vi "Read Script.vi"(2 "commands":string, 3 "script name":string) -> (0 "text from file":string, 1 "output array":dbl[][](array[numeric]))   [LabVIEW 2014]
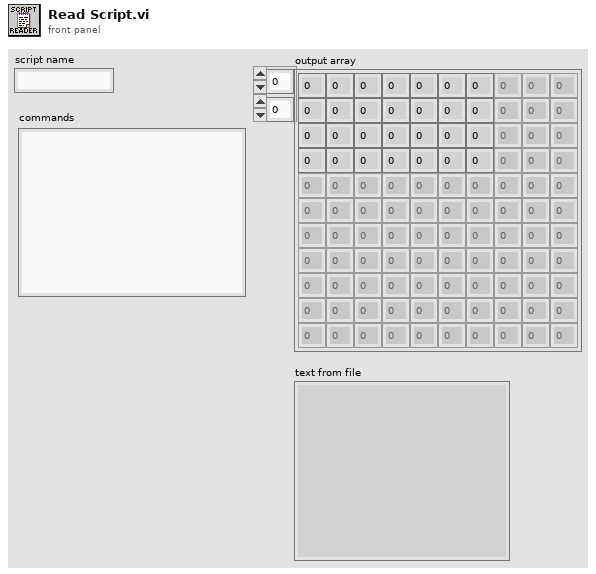
[diagram p1: front panel]
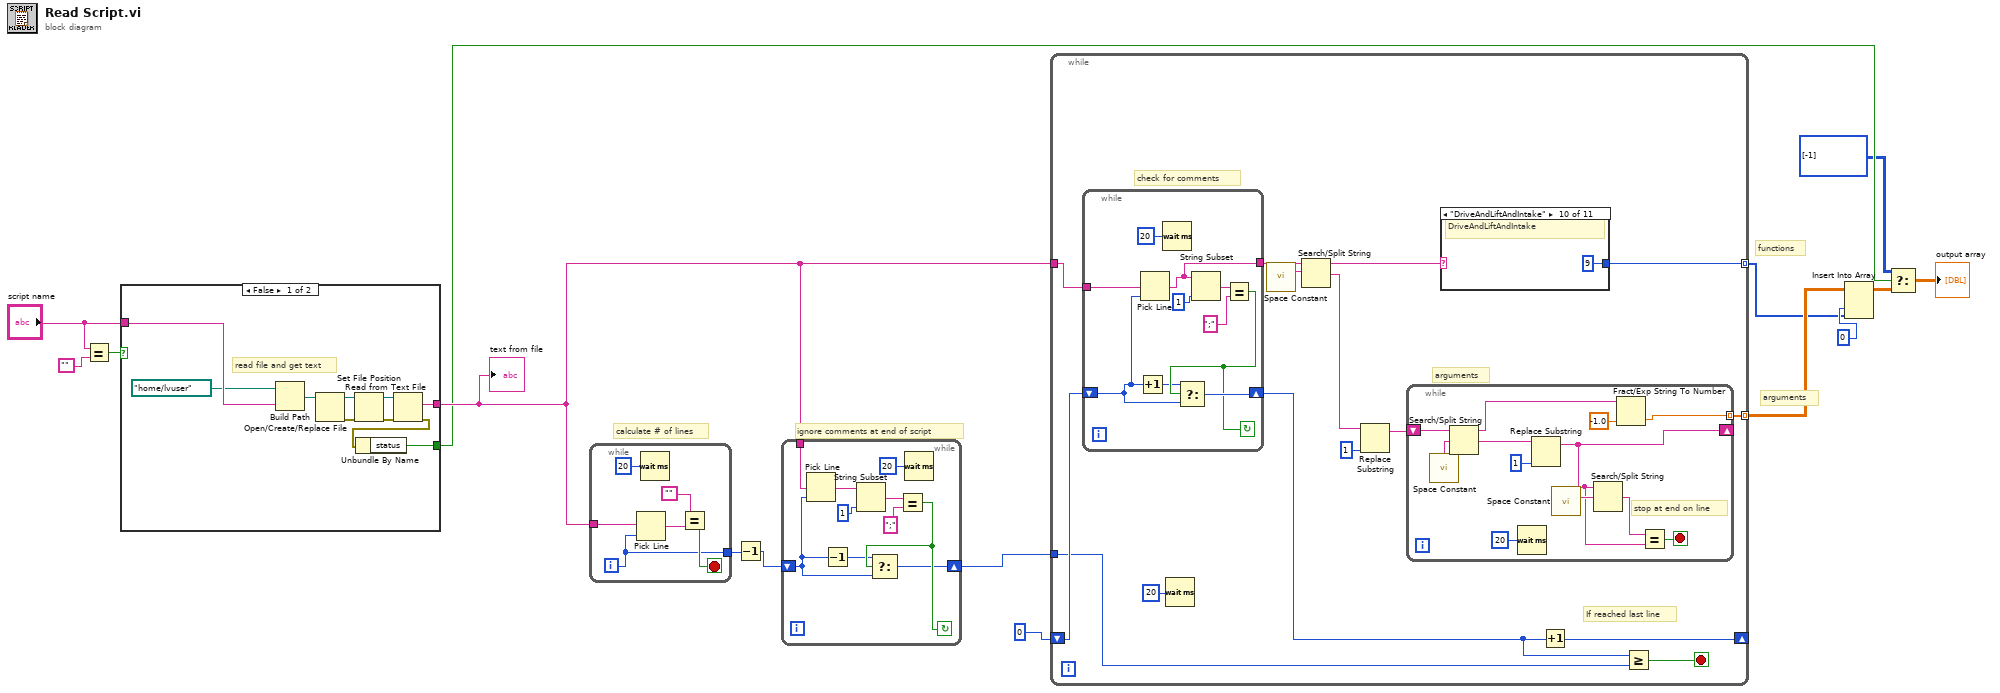
[diagram p0: block diagram]
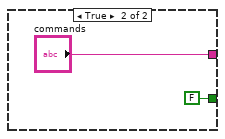
[diagram p2: hidden frame]
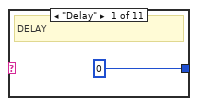
[diagram p3: hidden frame]
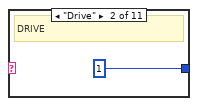
[diagram p4: hidden frame]
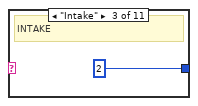
[diagram p5: hidden frame]
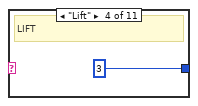
[diagram p6: hidden frame]
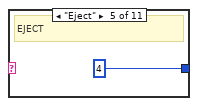
[diagram p7: hidden frame]
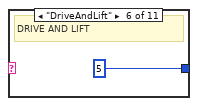
[diagram p8: hidden frame]
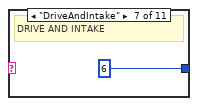
[diagram p9: hidden frame]
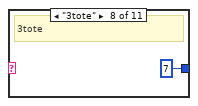
[diagram p10: hidden frame]
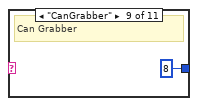
[diagram p11: hidden frame]
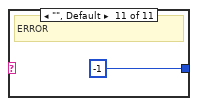
[diagram p12: hidden frame]
diagram:
  # "ignore comments at end of script"
  # "calculate # of lines"
  # "arguments"
  # "functions"
  n1 = Equal?(x="script name", y="") -> (x = y?=w6:bool)
  n2 = case shown="False" w6 {
    tunnel: "script name" -> [w22 _]
    tunnel: [w21 "commands"] -> w12
    tunnel: [w18 FALSE ("status")] -> w3
    frame False {
      # "read file and get text"
      n3 = Build Path(base path=path "/home/lvuser" ("configuration file path"), name or relative path=w22) -> (appended path=w23:path)
      n4 = Open/Create/Replace File(file path (use dialog)=w23) -> (refnum out=w25:refnum<file>, error out=w19:errorcluster)  [unwired: 5 in, 1 out]
      n5 = Set File Position(refnum=w25, error in=w19) -> (refnum out=w24:refnum<file>, error out=w20:errorcluster)  [unwired: 2 in]
      n6 = Read from Text File(file (use dialog)=w24, error in=w20) -> (text=w21:string, error out=w17:errorcluster)  [unwired: 2 in, 2 out]
      n7 = Unbundle By Name(w17) -> ("status"=w18:bool)
    }
    frame True {
    }
  }
  "text from file" <- w12
  n8 = while {
    tunnel: w12 -> [w33]
    tunnel: [w29] -> w10
    i -> [w29]
    stop <- w30 stop-if-true
    n9 = Pick Line(multi-line string=w33, line index=w29) -> (output string=w32:string)  [unwired: 1 in]
    n10 = Wait (ms)(milliseconds to wait=u32 20) -> ()  [unwired: 1 out]
    n11 = Equal?(x="", y=w32) -> (x = y?=w30:bool)
  }
  n12 = Decrement(x=w10) -> (x-1=w9:i32)
  n13 = while {
    tunnel: w12 -> [w43]
    shift-right: [w36] -> w11
    shift-left: w9 -> [w35]
    stop <- w38 continue-if-true
    n14 = Pick Line(multi-line string=w43, line index=w35) -> (output string=w41:string)  [unwired: 1 in]
    n15 = Decrement(x=w35) -> (x-1=w37:i32)
    n16 = String Subset(string=w41, length (rest)=1 ("length (rest)")) -> (substring=w40:string)  [unwired: 1 in]
    n17 = Equal?(x=w40, y=";") -> (x = y?=w38:bool)
    n18 = Select(t=w37, s=w38, f=w35) -> (s? t:f=w36:i32)
    n19 = Wait (ms)(milliseconds to wait=u32 20) -> ()  [unwired: 1 out]
  }
  n20 = while {
    tunnel: w12 -> [w51]
    tunnel: [w57] -> w14 mode=indexing
    shift-right: [w48] -> _
    shift-left: 0 -> [w53]
    tunnel: w11 -> [w49]
    tunnel: [w45] -> w1 mode=indexing
    stop <- w50 stop-if-true
    # "arguments"
    # "If reached last line"
    # "check for comments"
    n21 = while {
      tunnel: w51 -> [w79]
      tunnel: [w75] -> w52
      shift-right: [w74] -> w47
      shift-left: w53 -> [w71]
      stop <- w73 continue-if-true
      n22 = Increment(x=w71) -> (x+1=w72:i32)
      n23 = Pick Line(multi-line string=w79, line index=w71) -> (output string=w75:string)  [unwired: 1 in]
      n24 = Wait (ms)(milliseconds to wait=u32 20) -> ()  [unwired: 1 out]
      n25 = String Subset(string=w75, length (rest)=1 ("length (rest)")) -> (substring=w77:string)  [unwired: 1 in]
      n26 = Equal?(x=w77, y=";") -> (x = y?=w73:bool)
      n27 = Select(t=w72, s=w73, f=w71) -> (s? t:f=w74:i32)
    }
    n28 = Wait (ms)(milliseconds to wait=u32 20) -> ()  [unwired: 1 out]
    n29 = call <vilib>:"Space Constant.vi"() -> ("String"=w58:string)
    n30 = Search/Split String(string=w52, search string/char (-)=w58) -> (substring before match=w46:string, match + rest of string=w56:string)  [unwired: 1 in, 1 out]
    n31 = Replace Substring(2:1 ("length (len. of substring)"), 5:w56) -> (1:w54:string)  [unwired: 2 in, 1 out]
    n32 = while {
      shift-right: [w82] -> _
      shift-left: w54 -> [w83]
      tunnel: [w86] -> w57 mode=indexing
      stop <- w90 stop-if-true
      # "stop at end on line"
      n33 = call <vilib>:"Space Constant.vi"() -> ("String"=w91:string)
      n34 = Search/Split String(string=w83, search string/char (-)=w91) -> (substring before match=w87:string, match + rest of string=w89:string)  [unwired: 1 in, 1 out]
      n35 = Wait (ms)(milliseconds to wait=u32 20) -> ()  [unwired: 1 out]
      n36 = Replace Substring(2:1 ("length (len. of substring)"), 5:w89) -> (1:w82:string)  [unwired: 2 in, 1 out]
      n37 = call <vilib>:"Space Constant.vi"() -> ("String"=w85:string)
      n38 = Search/Split String(string=w82, search string/char (-)=w85) -> (match + rest of string=w84:string)  [unwired: 1 in, 2 out]
      n39 = Fract/Exp String To Number(string=w87, default (0 dbl)=-1.0 ("default (0 DBL)")) -> (number=w86:dbl)  [unwired: 2 in, 1 out]
      n40 = Equal?(x=w84, y=w82) -> (x = y?=w90:bool)
    }
    n41 = case shown="\"DriveAndLiftAndIntake\"" w46 {
      tunnel: [0 1 2 3 4 5 6 7 8 9 -1] -> w45
      frame "Delay" {
        # "DELAY"
      }
      frame "Drive" {
        # "DRIVE"
      }
      frame "Intake" {
        # "INTAKE"
      }
      frame "Lift" {
        # "LIFT"
      }
      frame "Eject" {
        # "EJECT"
      }
      frame "DriveAndLift" {
        # "DRIVE AND LIFT"
      }
      frame "DriveAndIntake" {
        # "DRIVE AND INTAKE"
      }
      frame "3tote" {
        # "3tote"
      }
      frame "CanGrabber" {
        # "Can Grabber"
      }
      frame "DriveAndLiftAndIntake" {
        # "DriveAndLiftAndIntake"
      }
      frame "", Default {
        # "ERROR"
      }
    }
    n42 = Increment(x=w47) -> (x+1=w48:i32)
    n43 = Greater Or Equal?(x=w47, y=w49) -> (x >= y?=w50:bool)
  }
  n44 = Insert Into Array(array=w14, index (col)=0 ("disabled index (col)"), new element=w1) -> (w4:dbl[][])  [unwired: 1 in]
  n45 = Select(t=i32[][] [[-1]], s=w3, f=w4) -> (s? t:f=→"output array":dbl[][])
